vi "getDevicesListBox.vi"(8 "error in (no error)":errorcluster, 11 "reference":refnum<vi>) -> (0 "error out":errorcluster, 2 "Item Names":string[](array[string]), 3 "reference out":refnum<vi>)   [LabVIEW 2010]
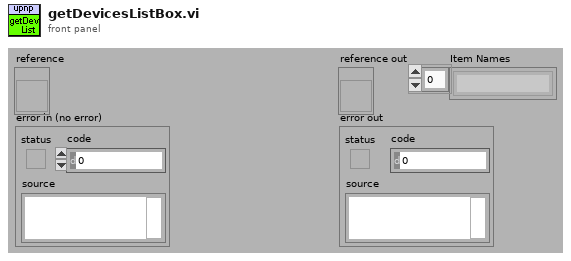
[diagram p1: front panel]
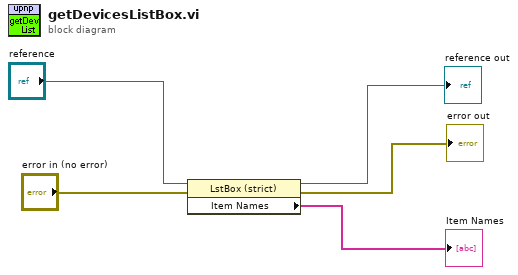
[diagram p0: block diagram]
diagram:
  n1 = property class="LstBox (strict)"(reference="reference", error in="error in (no error)") -> (reference out=→"reference out":refnum<vi>, error out=→"error out":errorcluster, "Item Names"=→"Item Names":string[])
